vi "平铺式顺序结构.vi"() -> ()   [LabVIEW 2022 SP3]
doc: "本VI是为《我和LabVIEW》一书编写的示例。\n关于本书的介绍请参考网页：\nhttp://ruanqizhen.spaces.live.com/blog/cns!5852D4F797C53FB6!4310.entry"
panel:
  out "用时 2":dbl caption="Time to Match" format="%.3f"
  out "当前数值 2":i32=5 caption="Current Number"
  in  "比较数值 2":i32=123 min=0 max=100000 step=1
  out "迭代次数 2":i32=124 caption="# of iterations"
  out "用时":dbl caption="Time to Match" format="%.3f"
  out "迭代次数":i32=124 caption="# of iterations"
  out "当前数值":i32=5 caption="Current Number"
  in  "比较数值":i32=123 min=0 max=100000 step=1
  # "sec"
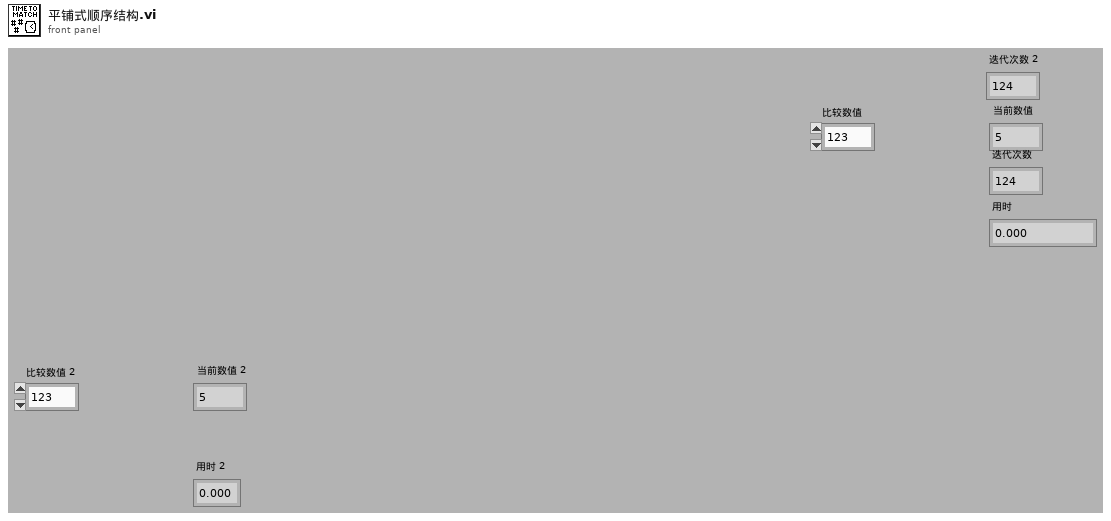
[diagram p1: front panel]
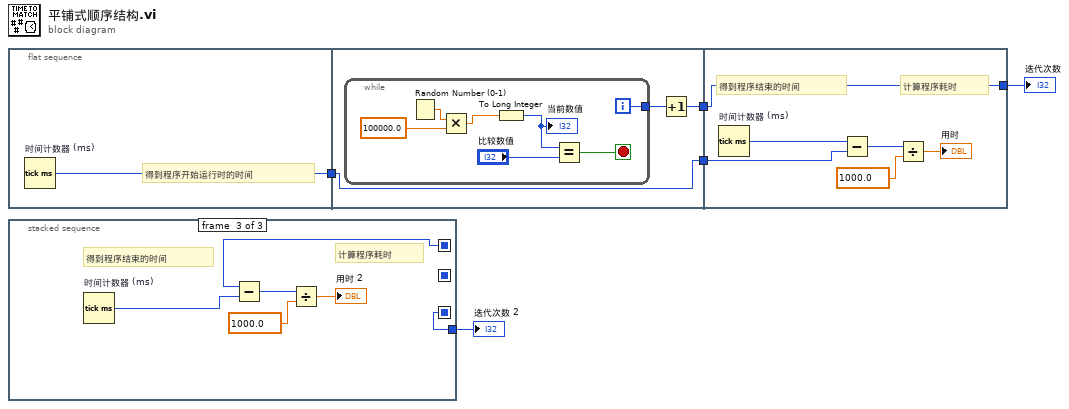
[diagram p0: block diagram]
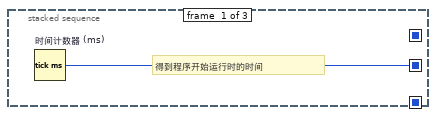
[diagram p2: hidden frame]
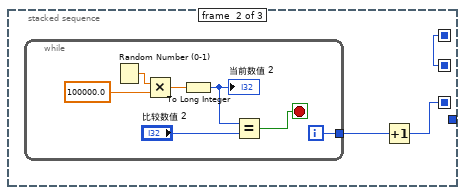
[diagram p3: hidden frame]
diagram:
  n1 = flat-sequence {
    tunnel: [w6] -> w4
    tunnel: w4 -> [w7]
    tunnel: [w8] -> w3
    tunnel: [w7] -> w2
    tunnel: [w17] -> w5
    tunnel: w3 -> [w17]
    tunnel: w2 -> [w18]
    frame #0 {
      # "得到程序开始运行时的时间"
      n2 = Tick Count (ms) "时间计数器 (ms)"() -> (millisecond timer value=w6:u32)
    }
    frame #1 {
      n3 = while {
        tunnel: [w11] -> w9
        i -> [w11]
        stop <- w12 stop-if-true
        n4 = Random Number (0-1)() -> (number: 0 to 1=w16:dbl)
        n5 = Multiply(x=w16, y=100000.0) -> (x*y=w14:dbl)
        n6 = To Long Integer(number=w14) -> (32bit integer=w10:i32)
        "当前数值" <- w10
        n7 = Equal?(x=w10, y="比较数值") -> (x = y?=w12:bool)
      }
      n8 = Increment(x=w9) -> (x+1=w8:i32)
    }
    frame #2 {
      # "计算程序耗时"
      # "得到程序结束的时间"
      n9 = Tick Count (ms) "时间计数器 (ms)"() -> (millisecond timer value=w22:u32)
      n10 = Subtract(x=w22, y=w18) -> (x-y=w21:u32)
      n11 = Divide(x=w21, y=1000.0) -> (x/y=→"用时":dbl)
    }
  }
  n12 = stacked-sequence {
    seq-local: [w23 _ _] -> [_ w24 _]
    seq-local: [_ w25 _] -> [_ _ w34]
    seq-local: [_ w24 _] -> [_ _ w35]
    tunnel: [_ _ w34] -> w1
    frame #0 {
      # "得到程序开始运行时的时间"
      n13 = Tick Count (ms) "时间计数器 (ms)"() -> (millisecond timer value=w23:u32)
    }
    frame #1 {
      n14 = while {
        tunnel: [w28] -> w26
        i -> [w28]
        stop <- w29 stop-if-true
        n15 = Random Number (0-1)() -> (number: 0 to 1=w33:dbl)
        n16 = Multiply(x=w33, y=100000.0) -> (x*y=w31:dbl)
        n17 = To Long Integer(number=w31) -> (32bit integer=w27:i32)
        "当前数值 2" <- w27
        n18 = Equal?(x=w27, y="比较数值 2") -> (x = y?=w29:bool)
      }
      n19 = Increment(x=w26) -> (x+1=w25:i32)
    }
    frame #2 {
      # "计算程序耗时"
      # "得到程序结束的时间"
      n20 = Tick Count (ms) "时间计数器 (ms)"() -> (millisecond timer value=w39:u32)
      n21 = Subtract(x=w35, y=w39) -> (x-y=w38:u32)
      n22 = Divide(x=w38, y=1000.0) -> (x/y=→"用时 2":dbl)
    }
  }
  "迭代次数 2" <- w1
  "迭代次数" <- w5
